vi "Load Image (16-bit) (UTF-8 Path).vi"(8 "error in (no error)":errorcluster, 11 "Path In":string) -> (0 "error out":errorcluster, 2 "Image (16-bit)":T1, 3 "Path Out":string)   [LabVIEW 2020, in "G-Image.lvlib"]
doc: "Load a 16-bit per channel image file from disk. The resulting image will be stored in a LabVIEW Picture style cluster, but uses a U16 array for the image data (instead of U8). This image data must be converted to U8 when displaying in a Picture control.\n\nIf the image being loaded isn't natively 16-bit per channel, it will be converted to 16-bit before being returned.\n\nSupported image types:\nPNG, JPEG, BMP, GIF, TGA, PSD, HDR, PIC, PNM\n\nWhen loading an animated GIF, only the first frame will be returned. Use <b>Load Animated GIF Image.vi</b> to read all frames."
uses:
  G-Image.lvlib
  Controls/Image 16-bit.ctl
  Private/Result To Error.vi
  <vilib>/Utility/error.llb/Error Cluster From Error Code.vi
  Private/Copy Image To Picture (16-bit).vi
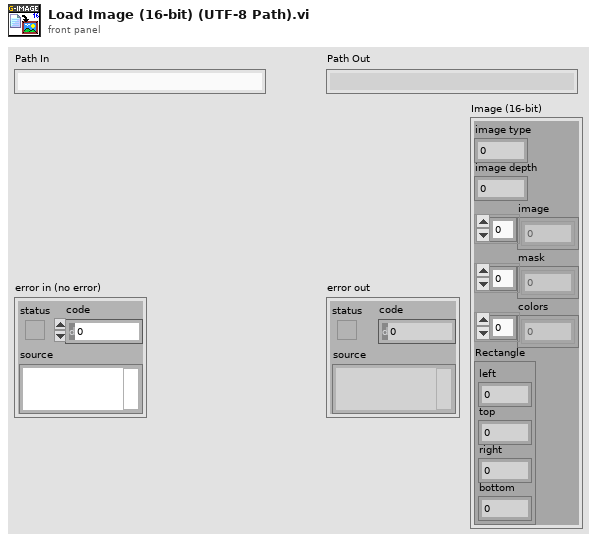
[diagram p1: front panel]
types:
  T1 = typedef "G-Image.lvlib/Image 16-bit.ctl" = cluster{"image type":i32, "image depth":i32, "image":u16[], "mask":u8[], "colors":u32[], "Rectangle":cluster{"left":i16, "top":i16, "right":i16, "bottom":i16}}
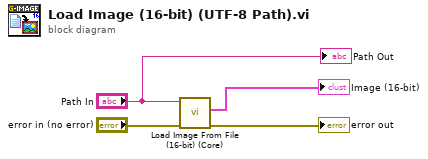
[diagram p0: block diagram]
diagram:
  n1 = call "Load Image From File (16-bit) (Core).vi"("error in (no error)"="error in (no error)", "Path In"="Path In") -> ("error out"=→"error out":errorcluster, "Image (16-bit)"=→"Image (16-bit)":T1)  [unwired: 7 in, 1 out]
  "Path Out" <- "Path In"
